vi "告警信息文本转换为协议i12031值.vi"(11 "字符串":string) -> (3 "十进制整型字符串":string)   [LabVIEW 2016, in "数据传输系统-05.lvlib"]
panel:
  out "匹配子字符串":string
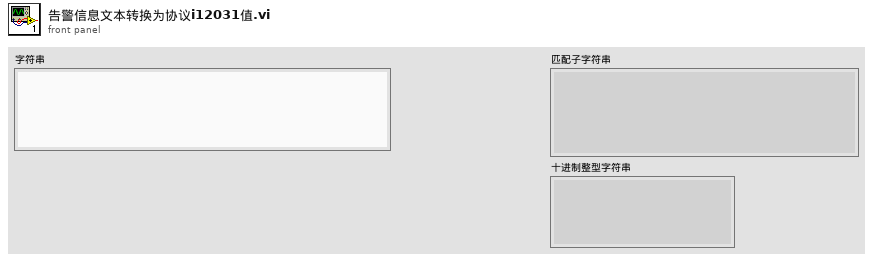
[diagram p1: front panel]
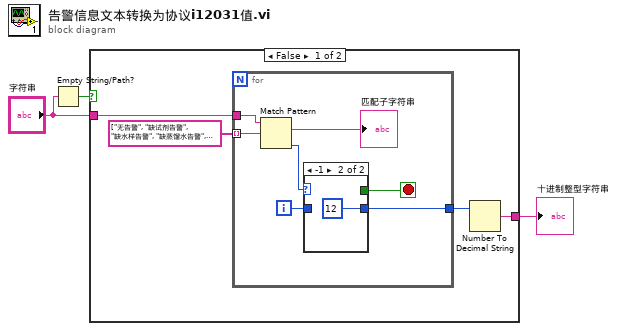
[diagram p0: block diagram]
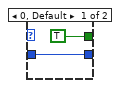
[diagram p2: hidden frame]
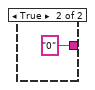
[diagram p3: hidden frame]
diagram:
  n1 = Empty String/Path?(string/path="字符串") -> (empty?=w1:bool)
  n2 = case shown="False" w1 {
    tunnel: "字符串" -> [w6 _]
    tunnel: [w4 "0"] -> w3
    frame False {
      n3 = for {
        tunnel: [w10] -> w5
        tunnel: string[] ["无告警", "缺试剂告警", "缺水样告警", "缺蒸馏水告警", "缺标液告警", "仪表漏液告警", "标定异常告警", "超量程告警", "加热异常", "低试剂预警", "超上限告警", "超下限告警", "仪表内部其他异常", "滴定异常告警", "电极异常告警", "量程切换告警", "参数设置告警", "PH电极电位异常", "电导率电极异常", "浊度光度异常", "溶解氧电极异常", "溶解氧光强异常"] -> [w9] mode=indexing
        tunnel: w6 -> [w8]
        i -> [w11]
        stop <- w12 stop-if-true
        n4 = Match Pattern(string=w8, regular expression=w9) -> (match substring=→"匹配子字符串":string, offset past match=w13:i32)  [unwired: 1 in, 2 out]
        n5 = case shown="-1" w13 {
          tunnel: [TRUE _] -> w12
          tunnel: w11 -> [w15 _]
          tunnel: [w15 12] -> w10
          frame 0, Default {
          }
          frame -1 {
          }
        }
      }
      n6 = Number To Decimal String(number=w5) -> (decimal integer string=w4:string)  [unwired: 1 in]
    }
    frame True {
    }
  }
  "十进制整型字符串" <- w3
